vi "XYGraph鼠标移动处理.vi"(6 "方框":refnum<vi>, 9 "开始坐标":T1, 10 "坐标":T1 caption="Coords", 11 "XYGraph":refnum<vi>) -> (2 "XY":cluster{"X":dbl, "Y":dbl}, 3 "XYGraph 2":refnum<vi>)   [LabVIEW 2018]
uses:
  <vilib>/Utility/miscctls.llb/LVPoint32TypeDef.ctl
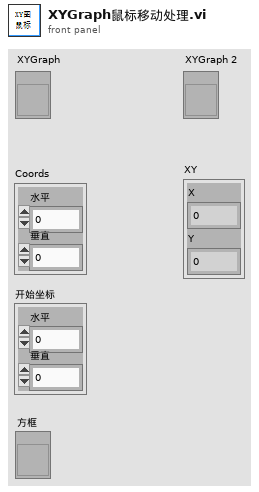
[diagram p1: front panel]
types:
  T1 = typedef "LVPoint32TypeDef.ctl" = cluster{"Horizontal":i32, "Vertical":i32}
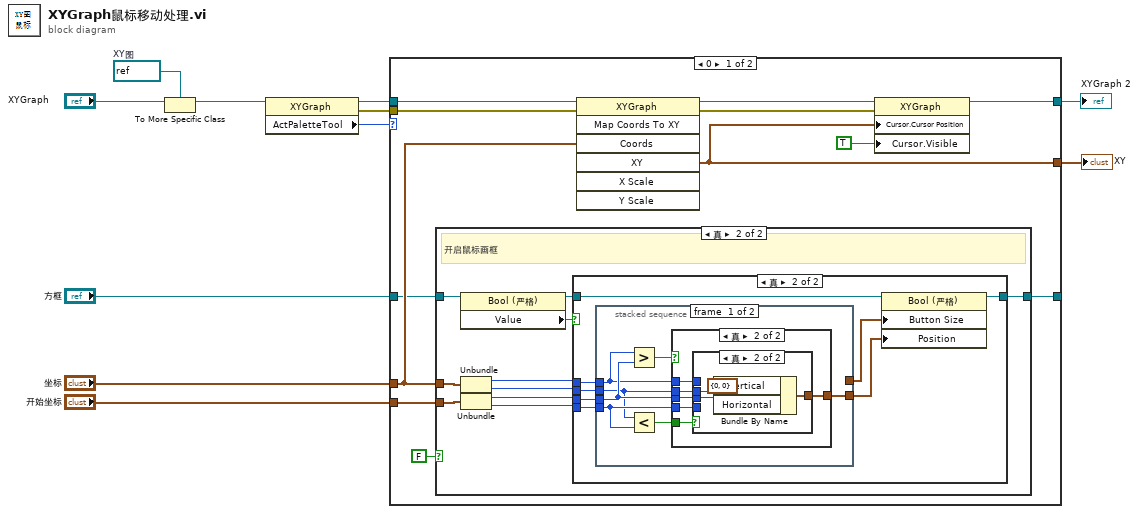
[diagram p0: block diagram]
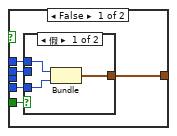
[diagram p4: hidden frame]
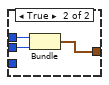
[diagram p5: hidden frame]
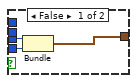
[diagram p6: hidden frame]
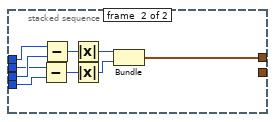
[diagram p7: hidden frame]
diagram:
  w2 = refnum<vi> refnum  # XY图
  n1 = To More Specific Class(target class=w2, reference="XYGraph") -> (specific class reference=w1:refnum<vi>)  [unwired: 1 in, 1 out]
  n2 = property class="XYGraph"(reference=w1) -> (reference out=w10:refnum<vi>, error out=w9:errorcluster, "ActPaletteTool"=w11:i32)  [unwired: 1 in]
  n3 = case shown="0" w11 {
    tunnel: w10 -> [w23 w85]
    tunnel: "坐标" -> [w17 _]
    tunnel: w9 -> [w20 _]
    tunnel: "开始坐标" -> [w18 _]
    tunnel: [w16 w84] -> _
    tunnel: [w15 w85] -> w4
    tunnel: "方框" -> [w14 w84]
    tunnel: [w12 _] -> w5
    frame 0 {
      n4 = case shown="真" FALSE {
        tunnel: w18 -> [_ w30]
        tunnel: w17 -> [_ w27]
        tunnel: [w24 w26] -> w16
        tunnel: w14 -> [w24 w25]
        frame False {
        }
        frame True {
          # "开启鼠标画框"
          n5 = property class="Bool (严格)"(reference=w25) -> (reference out=w28:refnum<vi>, "Value"=w29:bool)  [unwired: 1 in, 1 out]
          n6 = Unbundle(w27) -> ("Horizontal"=w34:i32, "Vertical"=w33:i32)
          n7 = Unbundle(w30) -> ("Horizontal"=w32:i32, "Vertical"=w31:i32)
          n8 = case shown="真" w29 {
            tunnel: w34 -> [_ w43]
            tunnel: w33 -> [_ w42]
            tunnel: w32 -> [_ w41]
            tunnel: w31 -> [_ w40]
            tunnel: w28 -> [w35 w39]
            tunnel: [w35 w36] -> w26
            frame False {
            }
            frame True {
              n9 = stacked-sequence {
                tunnel: w41 -> [w48 w80]
                tunnel: w40 -> [w47 w78]
                tunnel: w43 -> [w46 w81]
                tunnel: w42 -> [w45 w79]
                tunnel: [_ w75] -> w38
                tunnel: [w44 _] -> w37
                frame #0 {
                  n10 = Greater?(x=w46, y=w48) -> (0:w50:bool)
                  n11 = Less?(x=w45, y=w47) -> (x < y?=w49:bool)
                  n12 = case shown="真" w50 {
                    tunnel: w49 -> [w55 w67]
                    tunnel: w48 -> [_ w66]
                    tunnel: w47 -> [w54 w65]
                    tunnel: w46 -> [w53 w64]
                    tunnel: w45 -> [w51 w63]
                    tunnel: [w52 w62] -> w44
                    frame False {
                      n13 = case shown="假" w55 {
                        tunnel: w54 -> [w58 _]
                        tunnel: w53 -> [w57 w61]
                        tunnel: [w56 w59] -> w52
                        tunnel: w51 -> [_ w60]
                        frame False {
                          n14 = Bundle("Horizontal"=w57, "Vertical"=w58) -> (w56:cluster{"Horizontal":i32, "Vertical":i32})  [unwired: 1 in]
                        }
                        frame True {
                          n15 = Bundle("Horizontal"=w61, "Vertical"=w60) -> (w59:cluster{"Horizontal":i32, "Vertical":i32})  [unwired: 1 in]
                        }
                      }
                    }
                    frame True {
                      n16 = case shown="真" w67 {
                        tunnel: w66 -> [w70 w73]
                        tunnel: w65 -> [w69 _]
                        tunnel: w64 -> [_ _]
                        tunnel: w63 -> [_ w72]
                        tunnel: [w68 w71] -> w62
                        frame False {
                          n17 = Bundle("Horizontal"=w70, "Vertical"=w69) -> (w68:cluster{"Horizontal":i32, "Vertical":i32})  [unwired: 1 in]
                        }
                        frame True {
                          n18 = Bundle By Name(cluster=cluster{"Horizontal":i32, "Vertical":i32} {"Horizontal"=0, "Vertical"=0} ("输出簇"), "Vertical"=w72, "Horizontal"=w73) -> (w71:cluster{"Horizontal":i32, "Vertical":i32})
                        }
                      }
                    }
                  }
                }
                frame #1 {
                  n19 = Subtract(x=w79, y=w78) -> (x-y=w82:i32)
                  n20 = Subtract(x=w81, y=w80) -> (x-y=w83:i32)
                  n21 = Absolute Value(x=w83) -> (abs(x)=w77:i32)
                  n22 = Absolute Value(x=w82) -> (abs(x)=w76:i32)
                  n23 = Bundle(w77, w76) -> (w75:cluster{i32, i32})  [unwired: 1 in]
                }
              }
              n24 = property class="Bool (严格)"(reference=w39, "Button Size"=w38, "Position"=w37) -> (reference out=w36:refnum<vi>)  [unwired: 1 in, 1 out]
            }
          }
        }
      }
      n25 = invoke class="XYGraph" method="Map Coords To XY"(reference=w23, error in=w20, "Coords"=w17) -> (reference out=w22:refnum<vi>, error out=w21:errorcluster, "XY"=w12:cluster{"X":dbl, "Y":dbl})  [unwired: 4 in, 4 out]
      n26 = property class="XYGraph"(reference=w22, error in=w21, "Cursor.Cursor Position"=w12, "Cursor.Visible"=TRUE ("游标.可见")) -> (reference out=w15:refnum<vi>)  [unwired: 1 out]
    }
    frame 1, Default {
    }
  }
  "XYGraph 2" <- w4
  "XY" <- w5
